vi "Read Acyclic Frames.vi"(8 "error in":errorcluster, 11 "channel ref in":refnum<k20>) -> (0 "error out":errorcluster, 2 "acyclic frames":T1[](array[typedef]), 3 "channel ref out":refnum<k20>)   [LabVIEW 2020, in "AIM MIL-STD 1553 Import.lvlib"]
uses:
  AIM MIL-STD 1553 Import.lvlib
  63c09041-237f-4242-b1ce-dfabe9147df5.vi
  Constants.vi
  <vilib>/xml/NI_XML.lvlib
  Shared/Acyclic Frame Definition.ctl
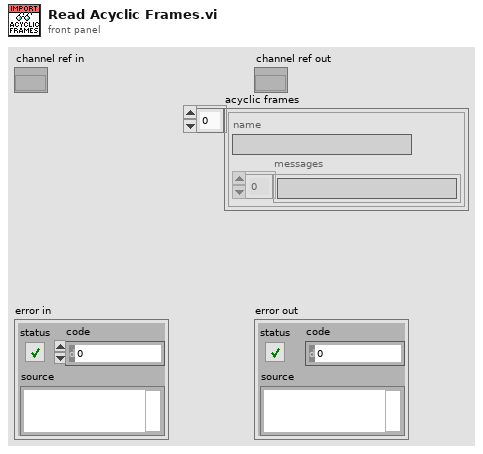
[diagram p1: front panel]
types:
  T1 = typedef "Acyclic Frame Definition.ctl" = cluster{"name":string, "messages":string[]}
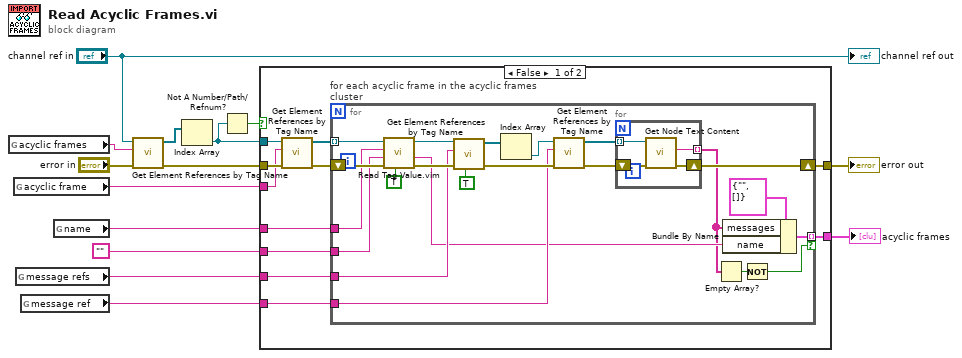
[diagram p0: block diagram]
diagram:
  n1 = global read "Constants.vi" "acyclic frames"() -> (w14:string)
  n2 = global read "Constants.vi" "acyclic frame"() -> (w4:string)
  n3 = global read "Constants.vi" "message refs"() -> (w3:string)
  n4 = global read "Constants.vi" "message ref"() -> (w2:string)
  n5 = global read "Constants.vi" "name"() -> (w10:string)
  n6 = call "Get Element References by Tag Name.vi"("error in"="error in", "tag name"=w14, "node in"="channel ref in") -> ("error out"=w12:errorcluster, "array of elements"=w7:refnum<k20>[])  [unwired: 7 in]
  n7 = Index Array(array=w7) -> (element=w5:refnum<k20>)  [unwired: 1 in]
  n8 = Not A Number/Path/Refnum?(number/path/refnum=w5) -> (NaN/Path/Refnum?=w6:bool)
  n9 = case shown="False" w6 {
    tunnel: [w25 w52] -> w13
    tunnel: w12 -> [w22 w52]
    tunnel: w10 -> [w24 _]
    tunnel: "" -> [w23 _]
    tunnel: w5 -> [w21 _]
    tunnel: w4 -> [w18 _]
    tunnel: w3 -> [w17 _]
    tunnel: w2 -> [w16 _]
    tunnel: [w15 _] -> w1
    frame False {
      n10 = call "Get Element References by Tag Name.vi"("error in"=w22, "tag name"=w18, "node in"=w21) -> ("error out"=w20:errorcluster, "array of elements"=w19:refnum<k20>[])  [unwired: 7 in]
      n11 = for "for each acyclic frame in the acyclic frames cluster" {
        shift-right: [w29] -> w25
        shift-left: w20 -> [w47]
        tunnel: w24 -> [w46]
        tunnel: w23 -> [w45]
        tunnel: w19 -> [w44] mode=indexing
        tunnel: w17 -> [w36]
        tunnel: w16 -> [w35]
        tunnel: [w30] -> w15 mode=indexing if=w26
        n12 = call "Read Tag Value.vim"("required (F)"=TRUE, "error in"=w47, "default"=w45, "tag name"=w46, "node in"=w44) -> ("error out"=w42:errorcluster, "value"=w31:string, "node out"=w41:refnum<k20>)  [unwired: 4 in]
        n13 = call "Get Element References by Tag Name.vi"("required (F)"=TRUE, "error in"=w42, "tag name"=w36, "node in"=w41) -> ("error out"=w38:errorcluster, "array of elements"=w40:refnum<k20>[])  [unwired: 6 in]
        n14 = Index Array(array=w40) -> (element=w39:refnum<k20>)  [unwired: 1 in]
        n15 = call "Get Element References by Tag Name.vi"("error in"=w38, "tag name"=w35, "node in"=w39) -> ("error out"=w33:errorcluster, "array of elements"=w34:refnum<k20>[])  [unwired: 7 in]
        n16 = for {
          tunnel: w34 -> [w51] mode=indexing
          shift-right: [w49] -> w29
          shift-left: w33 -> [w50]
          tunnel: [w48] -> w28 mode=indexing
          n17 = call <vilib>:"Get Node Text Content.vi"("error in (no error)"=w50, "node in"=w51) -> ("error out"=w49:errorcluster, "node text"=w48:string)  [unwired: 7 in, 1 out]
        }
        n18 = Empty Array?(array=w28) -> (empty?=w27:bool)
        n19 = Bundle By Name(cluster=T1 {"name"="", "messages"=[]} ("acyclic frame definition"), "messages"=w28, "name"=w31) -> (w30:T1)
        n20 = Not(x=w27) -> (.not. x?=w26:bool)
      }
    }
    frame True {
    }
  }
  "error out" <- w13
  "acyclic frames" <- w1
  "channel ref out" <- "channel ref in"
